vi "Main(170328).vi"() -> ()   [LabVIEW 2015]
uses:
  3jm module/3JM_mode.ctl
panel:
  in  "Save":bool
  out "XY 그래프":cluster{dbl[], dbl[]}(graph)
  in  "Stop":bool
  in  "VISA resource name":refnum<visa-resource-name> caption="Port"
  in  "Connection":bool
  out "문자열":string
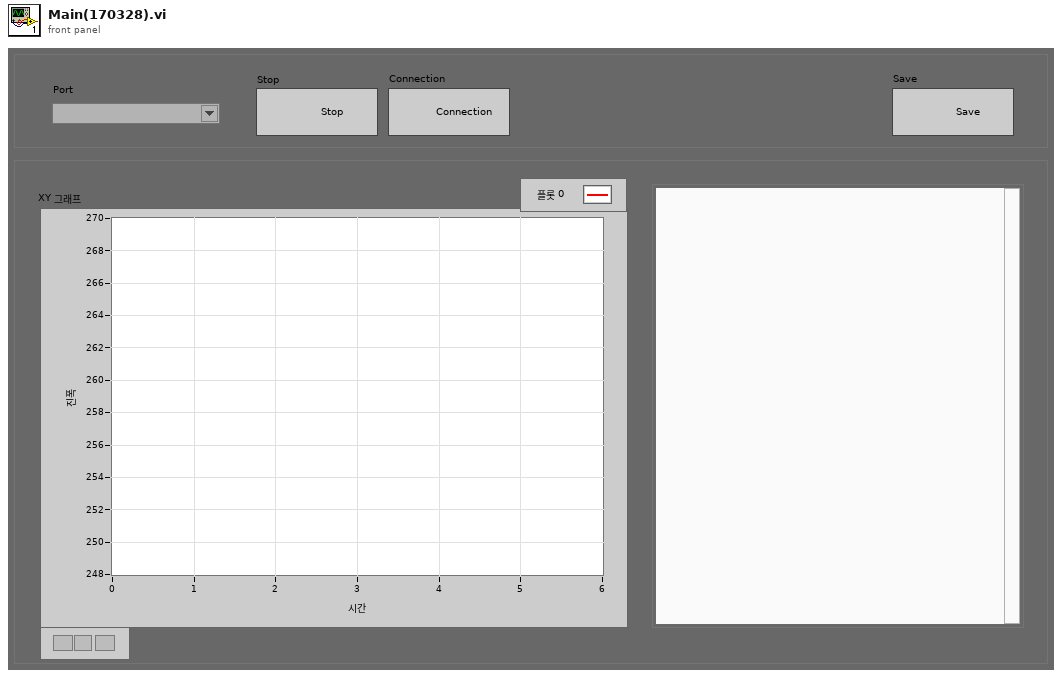
[diagram p1: front panel]
types:
  T1 = typedef "3JM_mode.ctl" = enum16{"Open", "Close", "Read"}
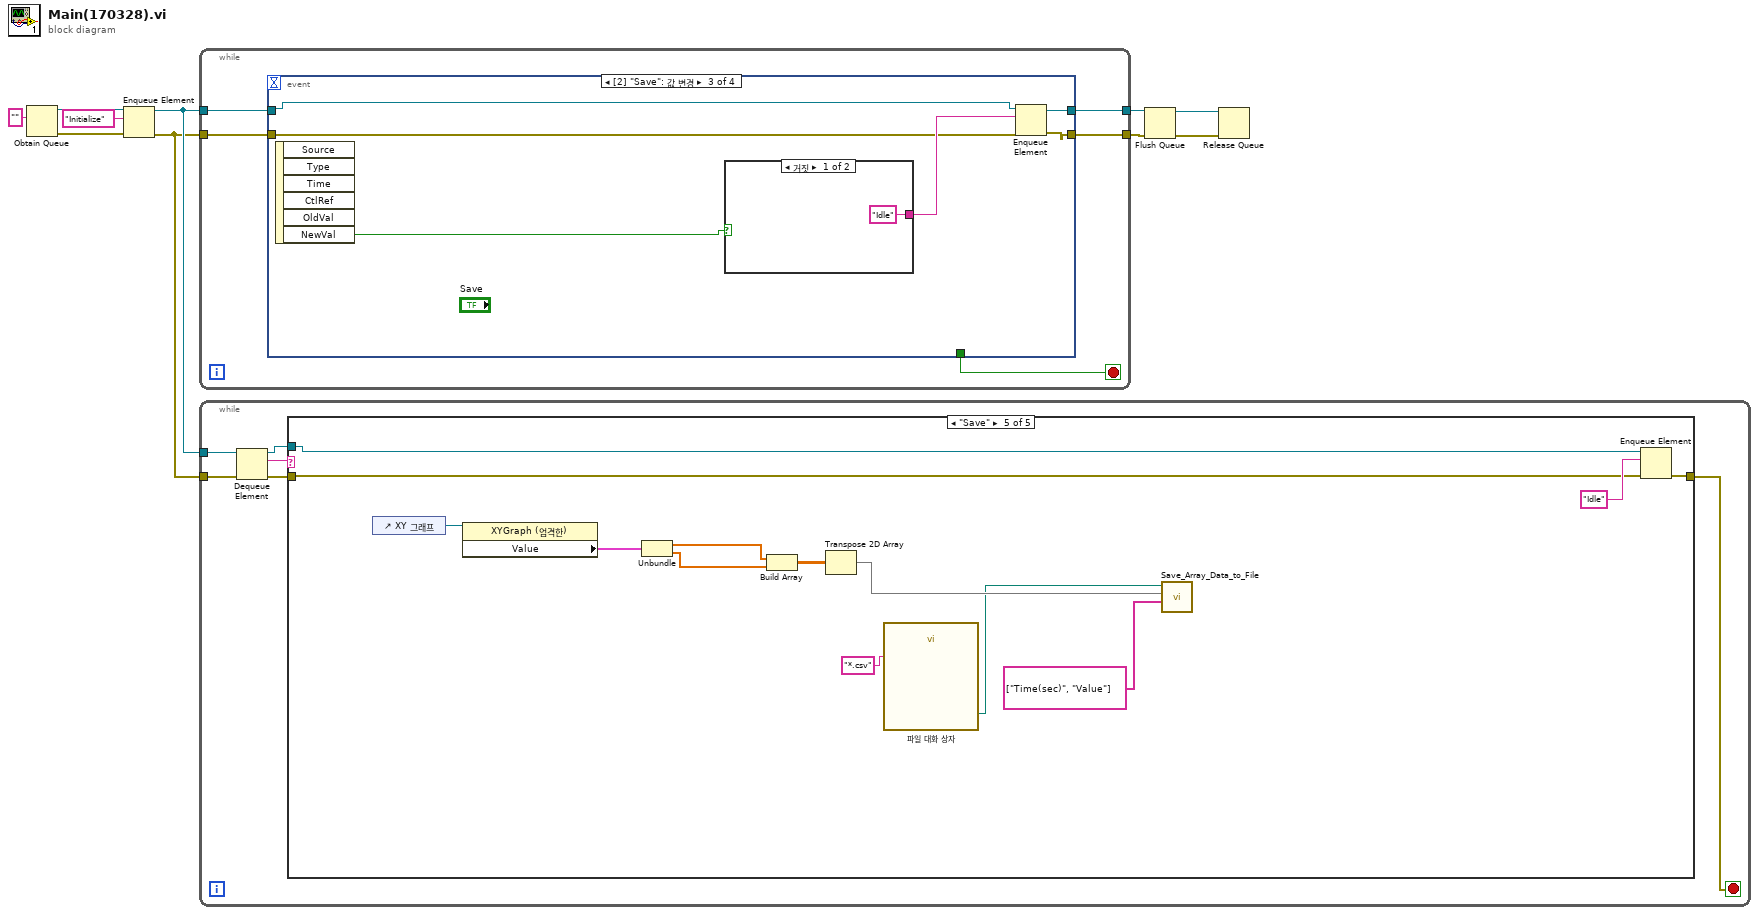
[diagram p0: block diagram]
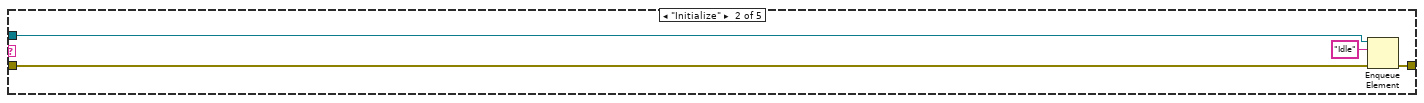
[diagram p3: hidden frame]
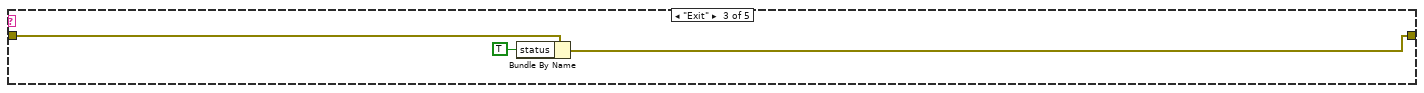
[diagram p4: hidden frame]
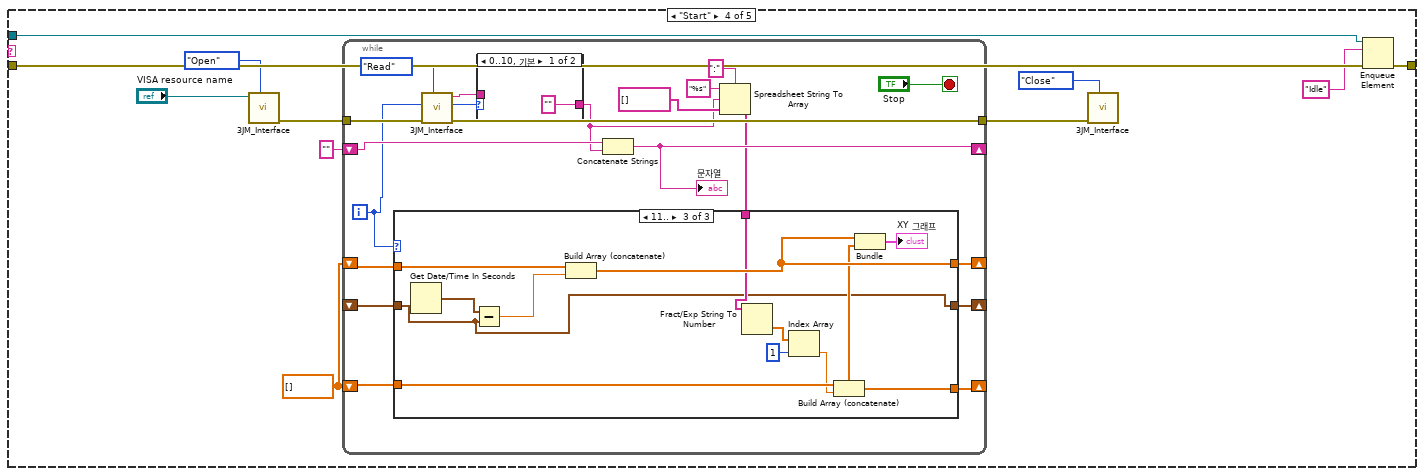
[diagram p5: hidden frame]
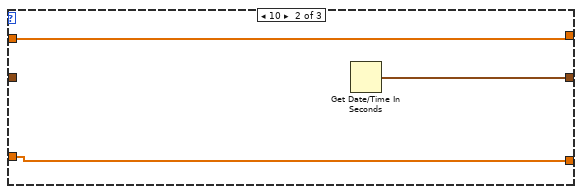
[diagram p7: hidden frame]
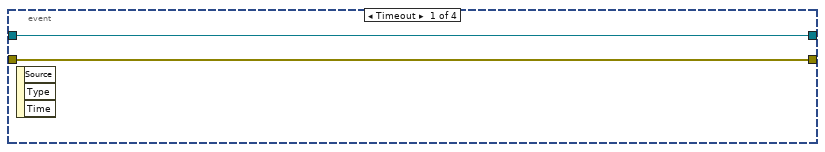
[diagram p9: hidden frame]
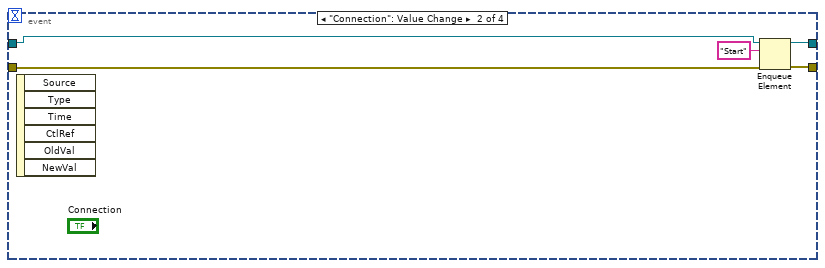
[diagram p10: hidden frame]
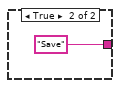
[diagram p11: hidden frame]
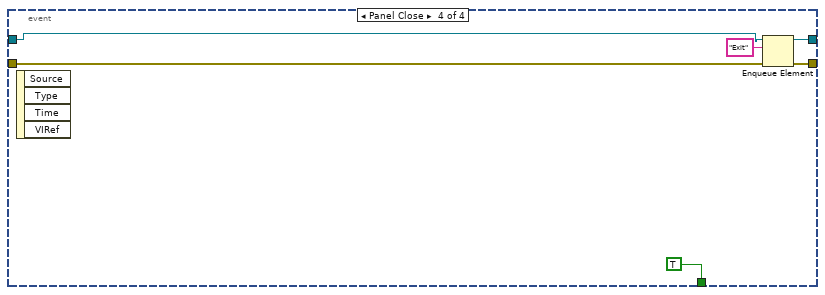
[diagram p12: hidden frame]
diagram:
  n1 = Obtain Queue(element data type="" ("element")) -> (queue out=w10:refnum<queue>, error out=w9:errorcluster)  [unwired: 4 in, 1 out]
  n2 = Enqueue Element(queue=w10, element="Initialize", error in (no error)=w9) -> (queue out=w2:refnum<queue>, error out=w1:errorcluster)  [unwired: 1 in, 1 out]
  n3 = while {
    tunnel: w2 -> [w15]
    tunnel: [w14] -> w4
    tunnel: w1 -> [w13]
    tunnel: [w12] -> w3
    stop <- w11 stop-if-true
    n4 = event shown="[2] \"Save\": 값 변경" {
      selector: _ -> [_ _ _ _]
      dyn-events: _ -> [_ _ _ _]
      timeout: _ -> [_ _ _ _]
      tunnel: w15 -> [w17 w19 w25 w31]
      tunnel: [w17 w20 w26 w33] -> w14
      tunnel: w13 -> [w16 w18 w24 w32]
      tunnel: [w16 w21 w27 w34] -> w12
      tunnel: [_ _ _ TRUE] -> w11
      event Timeout {
        n5 = event-data() -> ()  [unwired: 1 in, 3 out]
      }
      event "Connection": Value Change {
        n6 = event-data() -> ()  [unwired: 1 in, 6 out]
        n7 = Enqueue Element(queue=w19, element="Start", error in (no error)=w18) -> (queue out=w20:refnum<queue>, error out=w21:errorcluster)  [unwired: 1 in, 1 out]
      }
      event "Save": Value Change {
        n8 = event-data() -> ("NewVal"=w23:bool)  [unwired: 1 in, 5 out]
        n9 = case shown="거짓" w23 {
          tunnel: ["Idle" ("element") "Save" ("element")] -> w28
          frame False {
          }
          frame True {
          }
        }
        n10 = Enqueue Element(queue=w25, element=w28, error in (no error)=w24) -> (queue out=w26:refnum<queue>, error out=w27:errorcluster)  [unwired: 1 in, 1 out]
      }
      event Panel Close {
        n11 = event-data() -> ()  [unwired: 1 in, 4 out]
        n12 = Enqueue Element(queue=w31, element="Exit", error in (no error)=w32) -> (queue out=w33:refnum<queue>, error out=w34:errorcluster)  [unwired: 1 in, 1 out]
      }
    }
  }
  n13 = while {
    tunnel: w2 -> [w41]
    tunnel: w1 -> [w40]
    stop <- w37 stop-if-true
    n14 = Dequeue Element(queue=w41, error in (no error)=w40) -> (queue out=w38:refnum<queue>, element=w42:string, error out=w39:errorcluster)  [unwired: 1 in, 1 out]
    n15 = case shown="\"Save\"" w42 {
      tunnel: w39 -> [w43 w46 w50 w60 w111]
      tunnel: w38 -> [_ w45 _ w59 w110]
      tunnel: [w43 w44 w48 w61 w112] -> w37
      frame "Idle", Default {
      }
      frame "Initialize" {
        n16 = Enqueue Element(queue=w45, element="Idle", error in (no error)=w46) -> (error out=w44:errorcluster)  [unwired: 1 in, 2 out]
      }
      frame "Exit" {
        n17 = Bundle By Name(cluster=w50, "status"=TRUE) -> (w48:errorcluster)
      }
      frame "Start" {
        w51 = dbl[] []
        n18 = call "3JM_Interface.vi"("mode"=3JM_mode."Open", "VISA resource name"="VISA resource name") -> ("error out"=w55:errorcluster)  [unwired: 8 in, 1 out]
        n19 = while {
          tunnel: w55 -> [w79]
          tunnel: [w77] -> w53
          shift-right: [w67] -> _
          shift-left: "" -> [w75]
          shift-right: [w73] -> _
          shift-left: w51 -> [w74]
          shift-right: [w71] -> _
          shift-left: w51 -> [w72]
          shift-right: [w64] -> _
          shift-left: _ -> [w63]
          i -> [w70]
          stop <- "Stop" stop-if-true
          n20 = call "3JM_Interface.vi"("mode"=3JM_mode."Read", "error in (no error)"=w79) -> ("error out"=w77:errorcluster, "Read"=w76:string)  [unwired: 8 in]
          n21 = case shown="0..10, 기본" w70 {
            tunnel: w76 -> [_ w100]
            tunnel: ["" w100] -> w62
            frame 0..10, Default {
            }
            frame 11.. {
            }
          }
          n22 = Concatenate Strings(w75, w62) -> (w67:string)
          "문자열" <- w67
          n23 = Spreadsheet String To Array(delimiter (Tab)=":" ("구분 문자(탭)"), format string="%s" ("포맷 문자열"), spreadsheet string=w62, array type (2D Dbl)=string[] []) -> (array=w65:string[])
          n24 = case shown="11.." w70 {
            tunnel: w74 -> [w83 w85 w96]
            tunnel: [w83 w85 w95] -> w73
            tunnel: w72 -> [w82 w84 w94]
            tunnel: [w82 w84 w93] -> w71
            tunnel: w65 -> [_ _ w88]
            tunnel: [w81 w86 w87] -> w64
            tunnel: w63 -> [w81 _ w87]
            frame 0..9, Default {
            }
            frame 10 {
              n25 = Get Date/Time In Seconds() -> (seconds since 1Jan1904=w86:timestamp)
            }
            frame 11.. {
              n26 = Get Date/Time In Seconds() -> (seconds since 1Jan1904=w98:timestamp)
              n27 = Subtract(x=w98, y=w87) -> (x-y=w97:dbl)
              n28 = Build Array (concatenate)(w96, w97) -> (w95:dbl[])
              n29 = Fract/Exp String To Number(string=w88) -> (number=w91:dbl[])  [unwired: 3 in, 1 out]
              n30 = Index Array(array=w91, index=1 ("인덱스")) -> (element=w90:dbl)
              n31 = Build Array (concatenate)(w94, w90) -> (w93:dbl[])
              n32 = Bundle(w95, w93) -> (→"XY 그래프":cluster{dbl[], dbl[]})  [unwired: 1 in]
            }
          }
        }
        n33 = call "3JM_Interface.vi"("mode"=3JM_mode."Close", "error in (no error)"=w53) -> ()  [unwired: 8 in, 2 out]
        n34 = Enqueue Element(queue=w59, element="Idle", error in (no error)=w60) -> (error out=w61:errorcluster)  [unwired: 1 in, 2 out]
      }
      frame "Save" {
        n35 = control-ref of="XY 그래프"() -> (w109:refnum<vi>)
        n36 = property class="XYGraph (엄격한)"(reference=w109) -> ("Value"=w108:cluster{dbl[], dbl[]})  [unwired: 1 in, 2 out]
        n37 = Unbundle(w108) -> (w107:dbl[], w106:dbl[])
        n38 = Build Array(w107, w106) -> (w105:dbl[][])
        n39 = Transpose 2D Array(2D array=w105) -> (transposed array=w104:dbl[][])
        n40 = call "파일 대화 상자"("pattern (all files)"="*.csv" ("pattern label")) -> ("selected path"=w103:path)  [unwired: 11 in, 3 out]
        n41 = call "Save_Array_Data_to_File.vi"("Header Array"=string[] ["Time(sec)", "Value"], "Array"=w104, "file path (use dialog)"=w103) -> ()  [unwired: 8 in, 1 out]
        n42 = Enqueue Element(queue=w110, element="Idle", error in (no error)=w111) -> (error out=w112:errorcluster)  [unwired: 1 in, 2 out]
      }
    }
  }
  n43 = Flush Queue(queue=w4, error in (no error)=w3) -> (queue out=w6:refnum<queue>, error out=w5:errorcluster)  [unwired: 1 out]
  n44 = Release Queue(queue=w6, error in (no error)=w5) -> ()  [unwired: 1 in, 3 out]
